vi "Read Chopper Frequency.vi"(0 "Session Handle in":T1, 11 "error in (no error)":errorcluster) -> (4 "Session Handle out":T1, 6 "Frequency":dbl, 8 "Finished Ramping?":bool, 10 "Error Code":string, 15 "error out":errorcluster)   [LabVIEW 2015, in "PAS.lvclass"]
uses:
  PAS.lvclass
  Typedefs/Session Handle.ctl
panel:
  out "Success?":bool
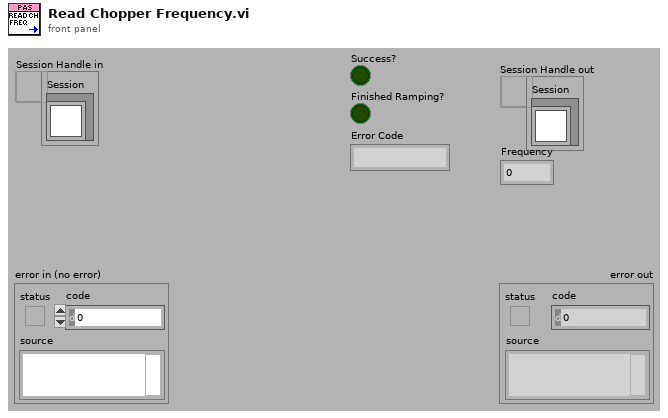
[diagram p1: front panel]
types:
  T1 = typedef "PAS.lvclass/Session Handle.ctl" = refnum<data-value>
  T2 = typedef "XNET Frame CAN.ctl" = cluster{"timestamp":timestamp, "payload":u8[], "identifier":u32, "type":T3, "extended?":bool, "echo?":bool}
  T3 = typedef "XNET Frame Type CAN.ctl" = u8
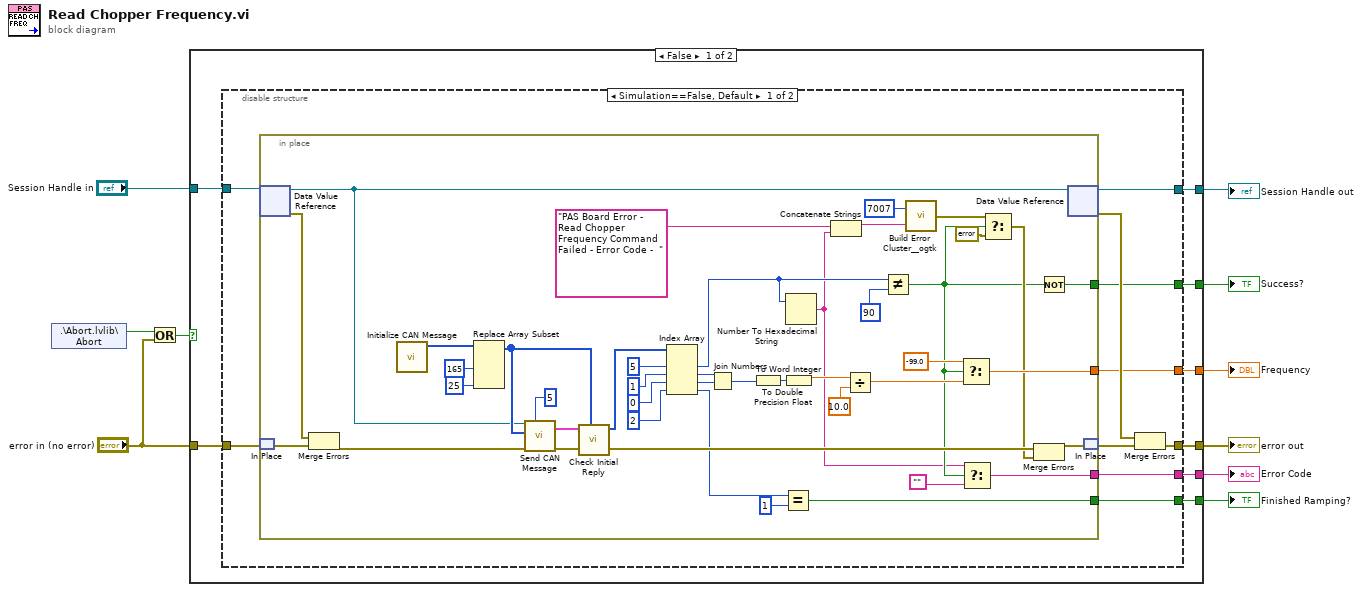
[diagram p0: block diagram]
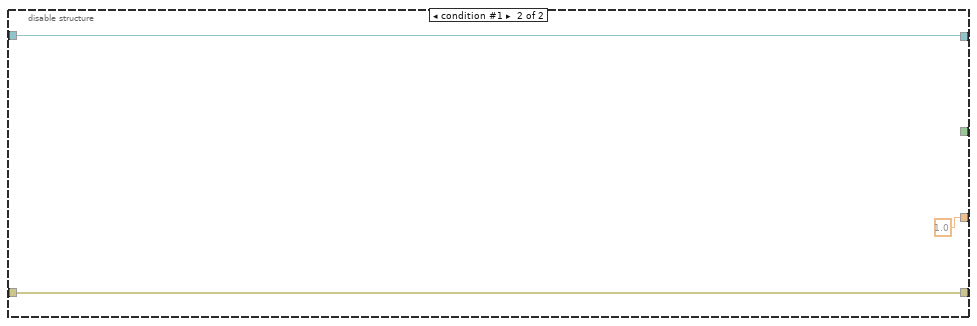
[diagram p2: hidden frame]
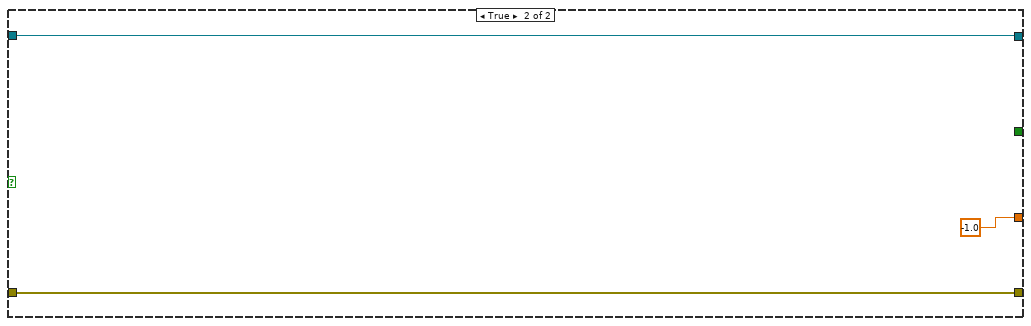
[diagram p3: hidden frame]
diagram:
  n1 = shared-variable ".\\Abort.lvlib\\Abort"() -> (w7:bool)  [unwired: 1 in, 1 out]
  n2 = Or(x=w7, y="error in (no error)") -> (x .or. y?=w5:bool)
  n3 = case shown="False" w5 {
    tunnel: [w18 w76] -> w9
    tunnel: [w17 w75] -> w8
    tunnel: "Session Handle in" -> [w16 w76]
    tunnel: "error in (no error)" -> [w15 w75]
    tunnel: [w14 -1.0] -> w4
    tunnel: [w13 _] -> w3
    tunnel: [w12 _] -> w2
    tunnel: [w11 _] -> w1
    frame False {
      n4 = disable-structure shown="Simulation==False, Default" {
        disable-tunnel: [w28 w73] -> w18
        disable-tunnel: [w25 w72] -> w17
        disable-tunnel: w16 -> [w24 w73]
        disable-tunnel: w15 -> [w23 w72]
        disable-tunnel: [w22 1.0] -> w14
        disable-tunnel: [w21 _] -> w13
        disable-tunnel: [w20 _] -> w12
        disable-tunnel: [w19 _] -> w11
        frame condition #0 (active) {
          n5 = in-place {
            in-place-border: [w43] -> w22
            in-place-border: [w54] -> w21
            in-place-border: [w33] -> w20
            in-place-border: [w29] -> w19
            n6 = in-place-dvr #1(w24) -> (w61:refnum<class "PAS.lvclass">, w66:errorcluster)
            n7 = in-place-match #2(w23) -> (w65:errorcluster)
            n8 = Merge Errors(w66, w65) -> (w60:errorcluster)
            n9 = call "Initialize CAN Message.vi"() -> ("Initial Payload"=w68:u8[])  [unwired: 11 in]
            n10 = Replace Array Subset(array=w68, new element #1=u8 165 ("new element/subarray"), new element #2=u8 25 ("new element/subarray")) -> (w64:u8[])  [unwired: 2 in]
            n11 = call "Send CAN Message.vi"("Number of Retries"=5, "error in (no error)"=w60, "payload"=w64, "Gas In"=w61) -> ("error out"=w38:errorcluster, "Reply"=w62:T2[])  [unwired: 5 in, 1 out]
            n12 = call "Check Initial Reply.vi"("Write Message"=w64, "Reply"=w62) -> ("Data Packet"=w67:u8[])  [unwired: 7 in, 2 out]
            n13 = Index Array(array=w67, index #1=5 ("index"), index #2=1 ("index"), index #3=0 ("index"), index #4=2 ("index")) -> (element #1=w55:u8, element #2=w50:u8, element #3=w49:u8, element #4=w35:u8)
            n14 = Join Numbers(hi=w50, lo=w49) -> ((hi.lo)=w48:u16)
            n15 = To Word Integer(number=w48) -> (16bit integer=w51:i16)
            n16 = Equal?(x=w35, y=u8 1) -> (x = y?=w33:bool)
            n17 = To Double Precision Float(number=w51) -> (double precision float=w45:dbl)
            n18 = Number To Hexadecimal String(2:w55) -> (0:w30:string)  [unwired: 1 in]
            n19 = Concatenate Strings("PAS Board Error -  Read Chopper Frequency Command Failed - Error Code -  " ("string"), w30) -> (w58:string)
            n20 = Divide(x=w45, y=10.0) -> (x/y=w40:dbl)
            n21 = Not Equal?(x=w55, y=u8 90 ("new element/subarray")) -> (x != y?=w31:bool)
            n22 = call <userlib>:"Build Error Cluster__ogtk.vi"("String to Prepend to source (\"\")"=w58, "code"=7007) -> ("error out"=w47:errorcluster)
            n23 = Select(t=-99.0, s=w31, f=w40) -> (s? t:f=w43:dbl)
            n24 = Select(t=w30, s=w31, f="") -> (s? t:f=w29:string)
            n25 = Select(t=w47, s=w31, f=errorcluster {"status"=FALSE, "code"=0, "source"=""}) -> (s? t:f=w37:errorcluster)
            n26 = Merge Errors(w38, w37) -> (w69:errorcluster)
            n27 = Not(x=w31) -> (.not. x?=w54:bool)
            n28 = in-place-dvr #1(w61) -> (w28:T1, w26:errorcluster)
            n29 = in-place-match #2(w69) -> (w27:errorcluster)
          }
          n30 = Merge Errors(w26, w27) -> (w25:errorcluster)
        }
        frame condition #1 {
        }
      }
    }
    frame True {
    }
  }
  "Session Handle out" <- w9
  "error out" <- w8
  "Frequency" <- w4
  "Success?" <- w3
  "Finished Ramping?" <- w2
  "Error Code" <- w1
